vi "Set Camera Mode Vision.vi"(1 "Set Camera Mode Message":T1={"type"="camera_mode", "Vision Mode"={"message"="vision", "Active?"=FALSE}, "Intake Mode"={"message"="intake", "Active?"=TRUE}}) -> (0 "Set Camera Mode Message":T1={"type"="camera_mode", "Vision Mode"={"message"="vision", "Active?"=TRUE}, "Intake Mode"={"message"="intake", "Active?"=FALSE}})   [LabVIEW 2016]
uses:
  Set Camera Mode Message.ctl
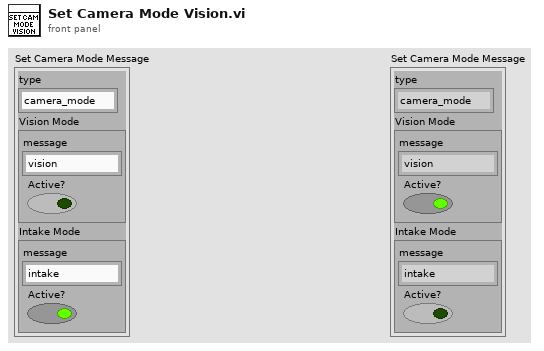
[diagram p1: front panel]
types:
  T1 = typedef "Set Camera Mode Message.ctl" = cluster{"type":string, "Vision Mode":cluster{"message":string, "Active?":bool}, "Intake Mode":cluster{"message":string, "Active?":bool}}
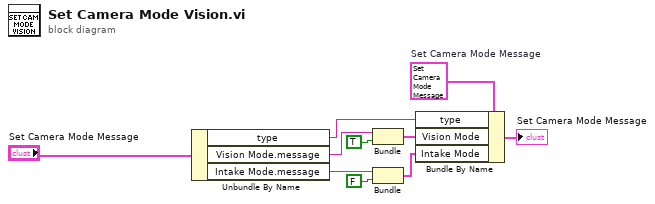
[diagram p0: block diagram]
diagram:
  w2 = T1 {"type"="camera_mode", "Vision Mode"={"message"="vision", "Active?"=TRUE}, "Intake Mode"={"message"="intake", "Active?"=FALSE}}  # Set Camera Mode Message
  n1 = Unbundle By Name("Set Camera Mode Message") -> ("type"=w10:string, "Vision Mode.message"=w9:string, "Intake Mode.message"=w6:string)
  n2 = Bundle("message"=w9, "Active?"=TRUE) -> (w7:cluster{"message":string, "Active?":bool})  [unwired: 1 in]
  n3 = Bundle("message"=w6, "Active?"=FALSE) -> (w4:cluster{"message":string, "Active?":bool})  [unwired: 1 in]
  n4 = Bundle By Name(cluster=w2, "type"=w10, "Vision Mode"=w7, "Intake Mode"=w4) -> (→"Set Camera Mode Message":T1)
